vi "Read.vi"(11 "SeqRunning Condition Config in":refnum<class "SeqRunning Condition Config.lvclass">) -> (3 "Sequence":string)   [LabVIEW 2020, in "VolatusSeqConfig.lvlib" / "SeqRunning Condition Config.lvclass"]
uses:
  SeqRunning Condition Config.lvclass
  SeqRunning Condition Config.lvclass/SeqRunning Condition Config.ctl
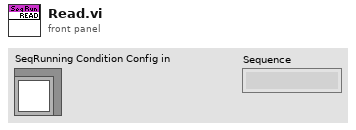
[diagram p1: front panel]
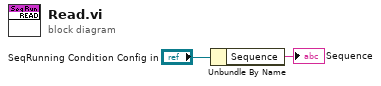
[diagram p0: block diagram]
diagram:
  n1 = Unbundle By Name("SeqRunning Condition Config in") -> ("Sequence"=→"Sequence":string)
